vi "Set Settings Element by Name__ogtk_TS.vi"(5 "element Name":string, 7 "index Array":i32[](array[numeric]), 8 "error in (no error)":errorcluster, 9 "Settings VData":variant[](array[variant]), 10 "New Element Value":variant, 11 "Cluster":variant) -> (0 "error out":errorcluster, 2 "Settings VData out":variant[](array[variant]))   [LabVIEW 2011]
doc: "Returns a cluster with element replaced with new element value. If <B>Element name</B> unwired, <B>New Element Value</B> data name is used. Data type of the new element is not checked for compatibility with replaced element."
panel:
  # "offset.Channel1.Value"
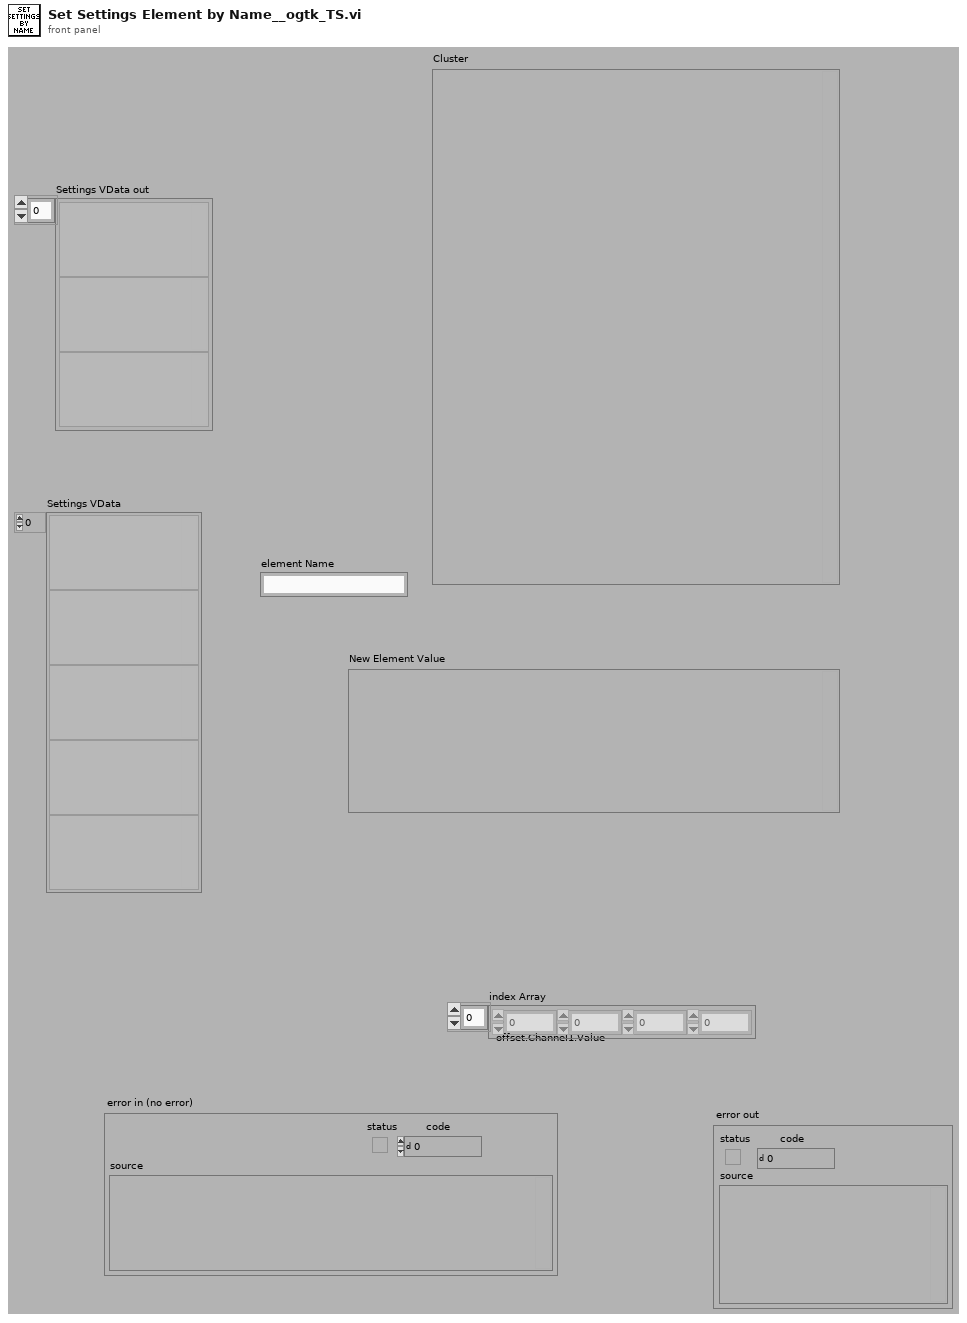
[diagram p1: front panel]
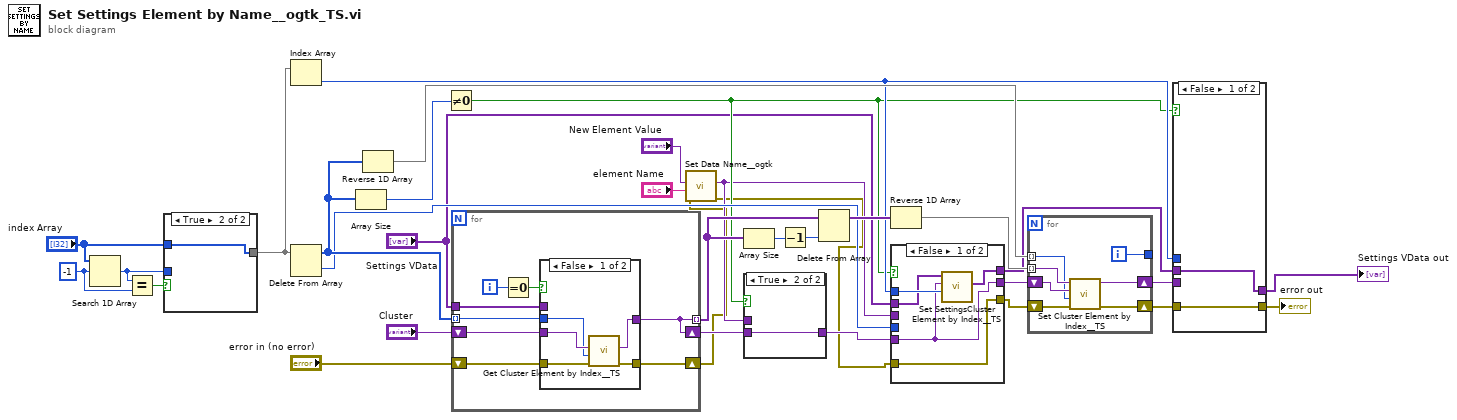
[diagram p0: block diagram]
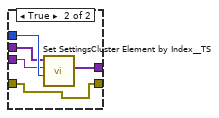
[diagram p2: hidden frame]
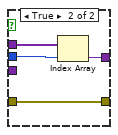
[diagram p3: hidden frame]
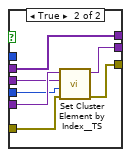
[diagram p4: hidden frame]
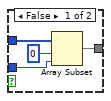
[diagram p6: hidden frame]
diagram:
  w24 = -1 ("element")
  n1 = Search 1D Array(1D array="index Array", element=w24) -> (index of element=w25:i32)  [unwired: 1 in]
  n2 = Equal?(x=w25, y=w24) -> (x = y?=w23:bool)
  n3 = case shown="True" w23 {
    tunnel: "index Array" -> [w37 w38]
    tunnel: w25 -> [w35 _]
    tunnel: [w34 w38] -> w15
    frame False {
      n4 = Array Subset(array=w37, index=0, length=w35) -> (w34:i32[])
    }
    frame True {
    }
  }
  n5 = Index Array(array=w15) -> (element=w14:i32)  [unwired: 1 in]
  n6 = Delete From Array(array=w15) -> (deleted portion=w20:i32, array with subset deleted=w22:i32[])  [unwired: 2 in]
  n7 = Array Size(array=w22) -> (size(s)=w21:i32)
  n8 = Reverse 1D Array(array=w22) -> (reversed array=w28:i32[])
  n9 = Not Equal To 0?(x=w21) -> (x != 0?=w13:bool)
  n10 = for {
    tunnel: w22 -> [w45] mode=indexing
    shift-right: [w44] -> w12
    shift-left: "Cluster" -> [w46]
    tunnel: [w44] -> w31 mode=indexing
    shift-right: [w43] -> w2
    shift-left: "error in (no error)" -> [w42]
    tunnel: "Settings VData" -> [w40]
    i -> [w41]
    n11 = Equal To 0?(x=w41) -> (x = 0?=w39:bool)
    n12 = case shown="False" w39 {
      tunnel: w46 -> [w51 _]
      tunnel: w45 -> [w50 w54]
      tunnel: [w49 w53] -> w44
      tunnel: [w48 w52] -> w43
      tunnel: w42 -> [w47 w52]
      tunnel: w40 -> [_ w55]
      frame False {
        n13 = call "Get Cluster Element by Index__TS.vi"("error in (no error)"=w47, "index of element"=w50, "Cluster"=w51) -> ("error out"=w48:errorcluster, "VElement"=w49:variant)  [unwired: 6 in, 1 out]
      }
      frame True {
        n14 = Index Array(array=w55, index=w54) -> (element=w53:variant)
      }
    }
  }
  n15 = call "Set Data Name__ogtk.vi"("error in (no error)"=w2, "Data Name"="element Name", "Data"="New Element Value") -> ("error out"=w1:errorcluster, "Renamed Data"=w10:variant)  [unwired: 7 in]
  n16 = Array Size(array=w31) -> (size(s)=w32:i32)
  n17 = case shown="True" w13 {
    tunnel: w12 -> [_ w57]
    tunnel: [w56 w57] -> w11
    tunnel: w10 -> [w56 _]
    frame False {
    }
    frame True {
    }
  }
  n18 = Decrement(x=w32) -> (x-1=w33:i32)
  n19 = Delete From Array(array=w31, index=w33) -> (array with subset deleted=w30:variant[])  [unwired: 1 in, 1 out]
  n20 = Reverse 1D Array(array=w30) -> (reversed array=w29:variant[])
  n21 = case shown="False" w13 {
    tunnel: w11 -> [w60 w69]
    tunnel: w10 -> [_ w68]
    tunnel: w20 -> [_ w67]
    tunnel: [w60 w66] -> w19
    tunnel: [w61 w65] -> w18
    tunnel: w1 -> [w61 w64]
    tunnel: "Settings VData" -> [w59 w63]
    tunnel: [w58 w63] -> w16
    tunnel: w14 -> [w62 _]
    frame False {
      n22 = call "Set SettingsCluster Element by Index__TS.vi"("index of element"=w62, "New Element Value"=w60, "Settings VData"=w59) -> ("Settings VData out"=w58:variant[])  [unwired: 7 in, 1 out]
    }
    frame True {
      n23 = call "Set Cluster Element by Index__TS.vi"("error in (no error)"=w64, "index of element"=w67, "New Element Value"=w68, "Cluster"=w69) -> ("error out"=w65:errorcluster, "VCluster out"=w66:variant)  [unwired: 5 in, 1 out]
    }
  }
  n24 = for {
    shift-right: [w71] -> w26
    shift-left: w19 -> [w74]
    tunnel: w29 -> [w75] mode=indexing
    tunnel: w28 -> [w73] mode=indexing
    shift-right: [w70] -> w27
    shift-left: w18 -> [w72]
    tunnel: [w76] -> _
    i -> [w76]
    n25 = call "Set Cluster Element by Index__TS.vi"("error in (no error)"=w72, "index of element"=w73, "New Element Value"=w74, "Cluster"=w75) -> ("error out"=w70:errorcluster, "VCluster out"=w71:variant)  [unwired: 5 in, 1 out]
  }
  n26 = case shown="False" w13 {
    tunnel: w14 -> [_ w83]
    tunnel: w26 -> [_ w82]
    tunnel: w27 -> [w78 w79]
    tunnel: [w78 w79] -> w3
    tunnel: w16 -> [w77 w81]
    tunnel: [w77 w80] -> w17
    frame False {
    }
    frame True {
      n27 = call "Set SettingsCluster Element by Index__TS.vi"("index of element"=w83, "New Element Value"=w82, "Settings VData"=w81) -> ("Settings VData out"=w80:variant[])  [unwired: 7 in, 1 out]
    }
  }
  "Settings VData out" <- w17
  "error out" <- w3
